vi "niDTS BT LE Tx Test Get Documentation.vi"(0 "Dummy Test Handle In":T1, 11 "error in (no error)":errorcluster) -> (4 "Dummy Test Handle Out":T1, 8 "Documentation":T2, 15 "error out":errorcluster)   [LabVIEW 2014, in "niDTS BT.lvlib"]
uses:
  niDTS BT.lvlib
  Framework/Test/Includes/niDTS Test INC Documentation.ctl
  Tx Test/Includes/niDTS BT Tx Test INC Handle.ctl
  Tx Test/Objects/BASE_class/niDTS BT Tx Test.lvclass
  Framework/niDTS Framework.lvlib
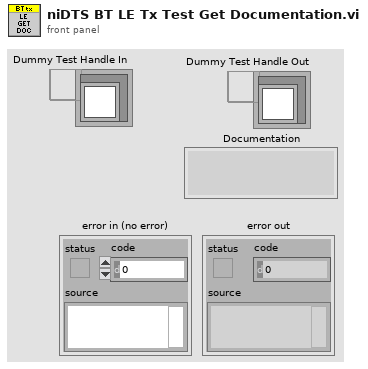
[diagram p1: front panel]
types:
  T1 = typedef "niDTS BT.lvlib/niDTS BT Tx Test INC Handle.ctl" = refnum<data-value>
  T2 = typedef "niDTS Framework.lvlib/niDTS Test INC Documentation.ctl" = string
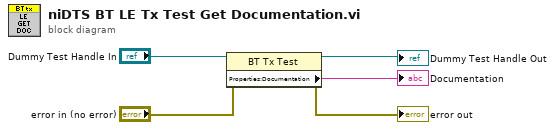
[diagram p0: block diagram]
diagram:
  n1 = property class="BT Tx Test"(reference="Dummy Test Handle In", error in="error in (no error)") -> (reference out=→"Dummy Test Handle Out":T1, error out=→"error out":errorcluster, "Properties:Documentation"=→"Documentation":T2)
